vi "Construct Notifier Transport.vi"() -> (0 "error out":errorcluster, 3 "NotifierTransport":refnum<class "NotifierTransport.lvclass">)   [LabVIEW 2020, in "NotifierTransport.lvclass"]
doc: "<License>\nCopyright © 2017 Composed Systems, LLC | All rights reserved\nwww.composed.io\n\nAuthor: Ethan Stern <ethan.stern@composed.io>\n\nThis software is provided \"AS IS\" WITHOUT WARRANTIES, either express or implied, AND IS FOR EDUCATIONAL PURPOSES ONLY.\n</License>"
uses:
  <vilib>/gpm_packages/@cs/transport/Source/Concrete/NotifierTransport/NotifierTransport.lvclass
  <vilib>/gpm_packages/@cs/transport/Source/Concrete/NotifierTransport/NotifierTransport.lvclass/NotifierTransport.ctl
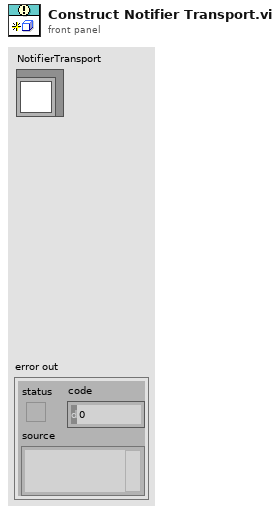
[diagram p1: front panel]
types:
  T1 = cluster{"Data":variant, "Publication Time":timestamp}
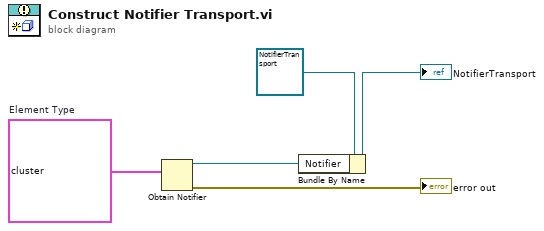
[diagram p0: block diagram]
diagram:
  w3 = T1 {"Data"=variant, "Publication Time"=timestamp(0 s since 1904-01-01)}  # Element Type
  n1 = Obtain Notifier(notification data type=w3) -> (notifier out=w1:refnum<notifier>, error out=→"error out":errorcluster)  [unwired: 3 in, 1 out]
  n2 = Bundle By Name(cluster=refnum<class "NotifierTransport.lvclass"> refnum ("QueueTransport.lvclass"), "Notifier"=w1) -> (→"NotifierTransport":refnum<class "NotifierTransport.lvclass">)
